vi "Set Routing Channel State Configurations.vi"(8 "error in":errorcluster, 10 "state configurations":T1, 11 "routing channel in":T4 format="%.0x") -> (0 "error out":errorcluster, 3 "routing channel out":T4=18446744073709551615 format="%.0x")   [LabVIEW 2020, in "Routing and Faulting Scripting.lvlib"]
doc: "Removes and replaces all existing states in a routing channel with the input."
uses:
  Routing and Faulting Scripting.lvlib
  <vilib>/NI VeriStand/Custom Device API/Custom Device Item Ref.ctl
  Shared/Channel States.ctl
  Shared/Routing State.ctl
  Shared/Connection.ctl
  NationalInstruments.VeriStand.SystemDefinitionAPI
  Constants/Scripting Constants.vi
  Utility/Connection to String.vi
  <vilib>/NI VeriStand/Custom Device API/Custom Device API.lvlib
  Shared/Routing and Faulting Shared.lvlib
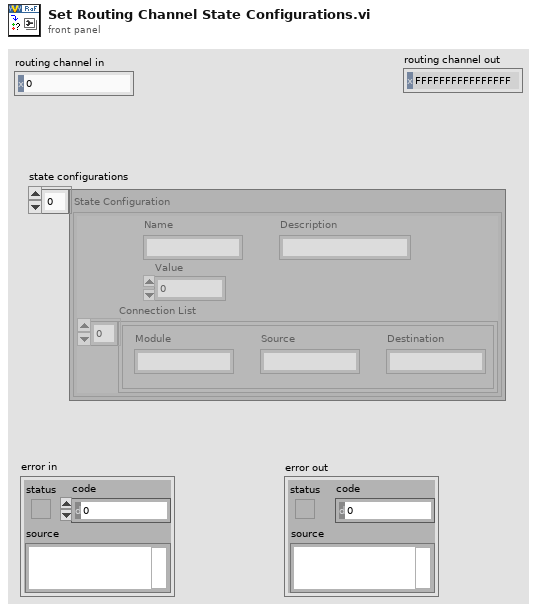
[diagram p1: front panel]
types:
  T1 = typedef "Routing and Faulting Shared.lvlib/Channel States.ctl" = T2[]
  T2 = typedef "Routing and Faulting Shared.lvlib/Routing State.ctl" = cluster{"Name":string, "Description":string, "Value":i32, "Connection List":T3[]}
  T3 = typedef "Routing and Faulting Shared.lvlib/Connection.ctl" = cluster{"Module":string, "Source":string, "Destination":string}
  T4 = typedef "Custom Device API.lvlib/Custom Device Item Ref.ctl" = u64
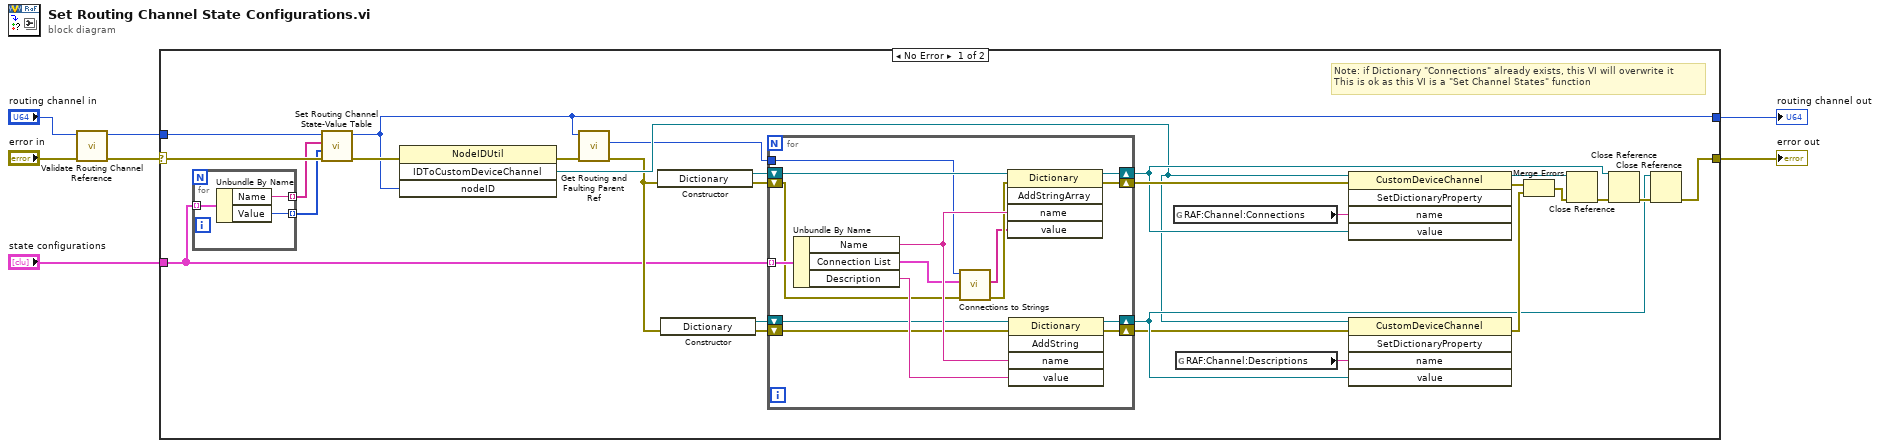
[diagram p0: block diagram]
diagram:
  n1 = call "Validate Routing Channel Reference.vi"("error in"="error in", "routing channel in"="routing channel in") -> ("error out"=w3:errorcluster, "routing channel out"=w1:T4)  [unwired: 8 in]
  n2 = case shown="No Error" w3 {
    selector: w3 -> [w13 w55]
    tunnel: [w35 w55] -> w6
    tunnel: w1 -> [w10 w54]
    tunnel: [w11 w54] -> w5
    tunnel: "state configurations" -> [w14 _]
    frame No Error {
      # "Note: if Dictionary \"Connections\" already exists, this VI will overwrite it\nThis is ok as this VI is a \"Set Channel States\" function"
      n3 = for {
        tunnel: w14 -> [w38] mode=indexing
        tunnel: [w37] -> w9 mode=indexing
        tunnel: [w36] -> w8 mode=indexing
        n4 = Unbundle By Name(w38) -> ("Name"=w37:string, "Value"=w36:i32)
      }
      n5 = call "Set Routing Channel State-Value Table.vi"("error in"=w13, "state values"=w8, "state names"=w9, "routing channel in"=w10) -> ("error out"=w12:errorcluster, "routing channel out"=w11:T4)  [unwired: 6 in]
      n6 = invoke class="NodeIDUtil" method="IDToCustomDeviceChannel"(error in=w12, "nodeID"=w11) -> (error out=w17:errorcluster, "IDToCustomDeviceChannel"=w18:refnum<k24>)  [unwired: 2 in, 2 out]
      n7 = call "Get Routing and Faulting Parent Ref.vi"("error in"=w17, "routing and faulting child in"=w11) -> ("error out"=w16:errorcluster, "routing and faulting"=w15:T4)  [unwired: 7 in, 1 out]
      n8 = constructor class="Dictionary"(error in=w16) -> (reference out=w32:refnum<k24>, error out=w20:errorcluster)  [unwired: 2 in, 1 out]
      n9 = constructor class="Dictionary"(error in=w16) -> (reference out=w31:refnum<k24>, error out=w21:errorcluster)  [unwired: 2 in, 1 out]
      n10 = for {
        tunnel: w14 -> [w53] mode=indexing
        shift-right: [w46] -> w28
        shift-left: w20 -> [w42]
        shift-right: [w50] -> w23
        shift-left: w31 -> [w48]
        shift-right: [w49] -> w24
        shift-left: w32 -> [w47]
        shift-right: [w45] -> w19
        shift-left: w21 -> [w43]
        tunnel: w15 -> [w39]
        n11 = Unbundle By Name(w53) -> ("Name"=w52:string, "Connection List"=w44:T3[], "Description"=w51:string)
        n12 = call "Connections to Strings.vi"("error in"=w42, "connection list"=w44, "routing and faulting in"=w39) -> ("error out"=w41:errorcluster, "connection strings"=w40:string[])  [unwired: 6 in, 1 out]
        n13 = invoke class="Dictionary" method="AddStringArray"(reference=w47, error in=w41, "name"=w52, "value"=w40) -> (reference out=w49:refnum<k24>, error out=w46:errorcluster)  [unwired: 1 in, 3 out]
        n14 = invoke class="Dictionary" method="AddString"(reference=w48, error in=w43, "name"=w52, "value"=w51) -> (reference out=w50:refnum<k24>, error out=w45:errorcluster)  [unwired: 1 in, 3 out]
      }
      n15 = global read "Scripting Constants.vi" "RAF:Channel:Connections"() -> (w33:string)
      n16 = global read "Scripting Constants.vi" "RAF:Channel:Descriptions"() -> (w22:string)
      n17 = invoke class="CustomDeviceChannel" method="SetDictionaryProperty"(reference=w18, error in=w28, "name"=w33, "value"=w24) -> (reference out=w34:refnum<k24>, error out=w26:errorcluster)  [unwired: 1 in, 3 out]
      n18 = invoke class="CustomDeviceChannel" method="SetDictionaryProperty"(reference=w18, error in=w19, "name"=w22, "value"=w23) -> (error out=w27:errorcluster)  [unwired: 1 in, 4 out]
      n19 = Merge Errors(w26, w27) -> (w25:errorcluster)
      n20 = Close Reference(reference=w34, error in (no error)=w25) -> (error out=w30:errorcluster)
      n21 = Close Reference(reference=w24, error in (no error)=w30) -> (error out=w29:errorcluster)
      n22 = Close Reference(reference=w23, error in (no error)=w29) -> (error out=w35:errorcluster)
    }
    frame Error {
    }
  }
  "routing channel out" <- w5
  "error out" <- w6
